vi "PPS Configure.vi"(8 "error in":errorcluster, 10 "Configure 2":T1={"Voltage Level (0.0 V)"=0.0, "CURRent Limit (0.0 A)"=0.0, "OVP LEVEL (0V)"=0.0, "OCP LEVEL (0A)"=0.0, "Enable OVP (T: Enable)"=TRUE, "Enable OCP (T: Enable)"=TRUE, "Enable Output "=TRUE, "Delays OCP"=0.0, "Delays OVP"=0.0, "Mode(0:Voltage)"=0, "CURRent Level (0.0 A)"=0.0, "Voltage Limit (0.0 V)"=0.0} {"Voltage Limit (0.0 V)" format="%.2f"; "Mode(0:Voltage)" items=["Voltage", "Current"]; "OCP LEVEL (0A)" format="%.2f"; "OVP LEVEL (0V)" format="%.2f"; "Voltage Level (0.0 V)" format="%.2f"}, 11 "IT-M3904D in":refnum<class "IT-M3904D.lvclass">) -> (0 "error out":errorcluster, 3 "IT-M3904D out":refnum<class "IT-M3904D.lvclass">)   [LabVIEW 2023, in "HardwareAbstractionLayer_LVOOP.lvlib" / "IT-M3904D.lvclass"]
uses:
  IT-M3904D.lvclass
  Control/PPS Configure Data.ctl
  <instrlib>/IT-M3900D/IT-M3900D.lvlib
  PowerSupply.lvclass
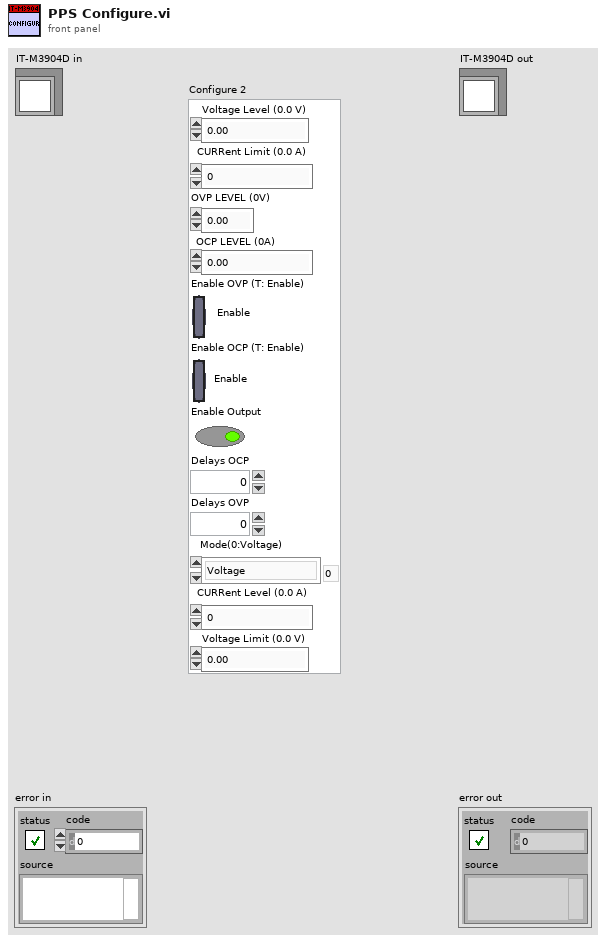
[diagram p1: front panel]
types:
  T1 = typedef "HardwareAbstractionLayer_LVOOP.lvlib/PowerSupply.lvclass/PPS Configure Data.ctl" = cluster{"Voltage Level (0.0 V)":dbl, "CURRent Limit (0.0 A)":dbl, "OVP LEVEL (0V)":dbl, "OCP LEVEL (0A)":dbl, "Enable OVP (T: Enable)":bool, "Enable OCP (T: Enable)":bool, "Enable Output ":bool, "Delays OCP":dbl, "Delays OVP":dbl, "Mode(0:Voltage)":u16, "CURRent Level (0.0 A)":dbl, "Voltage Limit (0.0 V)":dbl}
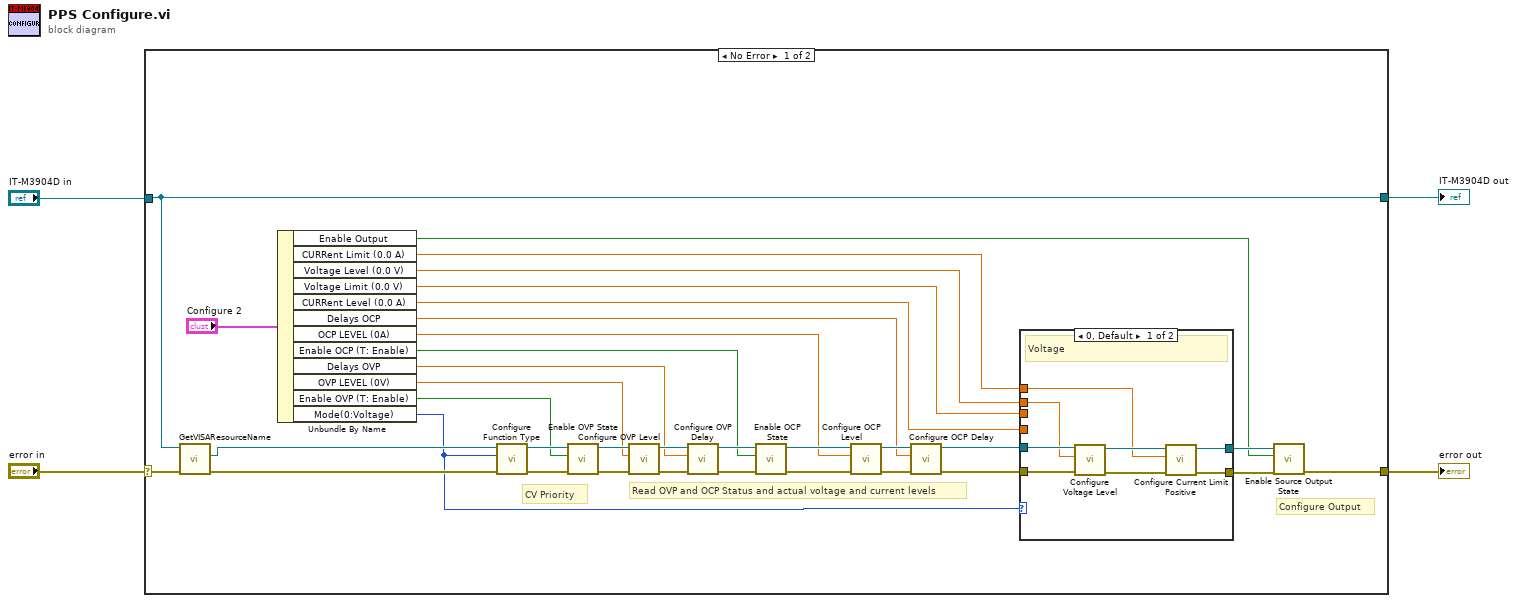
[diagram p0: block diagram]
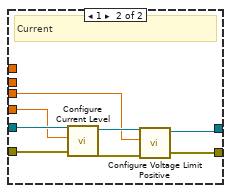
[diagram p2: hidden frame]
diagram:
  n1 = case shown="No Error" "error in" {
    selector: "error in" -> [w12 w55]
    tunnel: "IT-M3904D in" -> [w10 w56]
    tunnel: [w10 w56] -> w2
    tunnel: [w22 w55] -> w1
    frame No Error {
      # "CV Priority"
      # "Read OVP and OCP Status and actual voltage and current levels"
      # "Configure Output"
      n2 = call "GetVISAResourceName.vi"("error in (no error)"=w12, "object in"=w10) -> ("error out"=w11:errorcluster, "VISA resource name"=w9:refnum<visa-resource-name>)  [unwired: 7 in, 1 out]
      n3 = Unbundle By Name("Configure 2") -> ("Enable Output"=w13:bool, "CURRent Limit (0.0 A)"=w14:dbl, "Voltage Level (0.0 V)"=w15:dbl, "Voltage Limit (0.0 V)"=w7:dbl, "CURRent Level (0.0 A)"=w6:dbl, "Delays OCP"=w16:dbl, "OCP LEVEL (0A)"=w17:dbl, "Enable OCP (T: Enable)"=w18:bool, "Delays OVP"=w19:dbl, "OVP LEVEL (0V)"=w20:dbl, "Enable OVP (T: Enable)"=w21:bool, "Mode(0:Voltage)"=w8:u16)
      n4 = call <instrlib>:"Configure Function Type.vi"("error in"=w11, "Type"=w8, "VISA resource name"=w9) -> ("error out"=w37:errorcluster, "VISA resource name out"=w38:refnum<visa-resource-name>)  [unwired: 7 in]
      n5 = call <instrlib>:"Enable OVP State.vi"("error in"=w37, "State"=w21, "VISA resource name"=w38) -> ("error out"=w35:errorcluster, "VISA resource name out"=w36:refnum<visa-resource-name>)  [unwired: 7 in]
      n6 = call <instrlib>:"Configure OVP Level.vi"("error in"=w35, "Level(V)"=w20, "VISA resource name"=w36) -> ("error out"=w33:errorcluster, "VISA resource name out"=w34:refnum<visa-resource-name>)  [unwired: 7 in]
      n7 = call <instrlib>:"Configure OVP Delay.vi"("error in"=w33, "Delay(S)"=w19, "VISA resource name"=w34) -> ("error out"=w31:errorcluster, "VISA resource name out"=w32:refnum<visa-resource-name>)  [unwired: 7 in]
      n8 = call <instrlib>:"Enable OCP State.vi"("error in"=w31, "State"=w18, "VISA resource name"=w32) -> ("error out"=w29:errorcluster, "VISA resource name out"=w30:refnum<visa-resource-name>)  [unwired: 7 in]
      n9 = call <instrlib>:"Configure OCP Level.vi"("error in"=w29, "Level(A)"=w17, "VISA resource name"=w30) -> ("error out"=w27:errorcluster, "VISA resource name out"=w28:refnum<visa-resource-name>)  [unwired: 7 in]
      n10 = call <instrlib>:"Configure OCP Delay.vi"("error in"=w27, "Delay(S)"=w16, "VISA resource name"=w28) -> ("error out"=w25:errorcluster, "VISA resource name out"=w26:refnum<visa-resource-name>)  [unwired: 7 in]
      n11 = case shown="0, Default" w8 {
        tunnel: w26 -> [w46 w54]
        tunnel: w25 -> [w45 w53]
        tunnel: [w42 w50] -> w24
        tunnel: [w41 w49] -> w23
        tunnel: w15 -> [w40 _]
        tunnel: w14 -> [w39 _]
        tunnel: w7 -> [_ w47]
        tunnel: w6 -> [_ w48]
        frame 0, Default {
          # "Voltage"
          n12 = call <instrlib>:"Configure Voltage Level.vi"("error in"=w45, "Voltage(V)"=w40, "VISA resource name"=w46) -> ("error out"=w43:errorcluster, "VISA resource name out"=w44:refnum<visa-resource-name>)  [unwired: 7 in]
          n13 = call <instrlib>:"Configure Current Limit Positive.vi"("error in"=w43, "Value(A)"=w39, "VISA resource name"=w44) -> ("error out"=w41:errorcluster, "VISA resource name out"=w42:refnum<visa-resource-name>)  [unwired: 7 in]
        }
        frame 1 {
          # "Current"
          n14 = call <instrlib>:"Configure Current Level.vi"("error in"=w53, "Current(A)"=w48, "VISA resource name"=w54) -> ("error out"=w51:errorcluster, "VISA resource name out"=w52:refnum<visa-resource-name>)  [unwired: 7 in]
          n15 = call <instrlib>:"Configure Voltage Limit Positive.vi"("error in"=w51, "Limit(V)"=w47, "VISA resource name"=w52) -> ("error out"=w49:errorcluster, "VISA resource name out"=w50:refnum<visa-resource-name>)  [unwired: 7 in]
        }
      }
      n16 = call <instrlib>:"Enable Source Output State.vi"("error in"=w23, "State"=w13, "VISA resource name"=w24) -> ("error out"=w22:errorcluster)  [unwired: 7 in, 1 out]
    }
    frame Error {
    }
  }
  "error out" <- w1
  "IT-M3904D out" <- w2
